vi "Test Reset.vi"(11 "Error in":errorcluster) -> (15 "Error out":errorcluster)   [LabVIEW 2020, in "StopWatchTests.lvlib"]
doc: "This VI is used for validating reset button in stopwatch"
uses:
  StopWatchTests.lvlib
  <vilib>/SLL Drona/APIs/Stimulus/ControlValue/SetValueAuto.vi
  <vilib>/SLL Drona/APIs/Assert/AssertControlValue/Equal.vi
  <vilib>/SLL Drona/APIs/Assert/AssertControlValue/Greater.vi
  <vilib>/SLL Drona/APIs/Stimulus/VI/CloseVI.vi
  <vilib>/addons/_JKI Toolkits/Caraya/classes/Test/Test.lvclass
  <vilib>/SLL Drona/Drona.lvlib
  <vilib>/SLL Drona/APIs/Stimulus/ControlValue/ControlValue.lvlib
  <vilib>/SLL Drona/APIs/Assert/AssertControlValue/AssertControlValue.lvlib
  <vilib>/SLL Drona/APIs/Stimulus/VI/VI.lvlib
panel:
  # "RESET TEST"
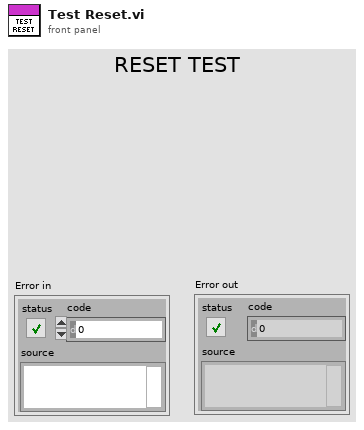
[diagram p1: front panel]
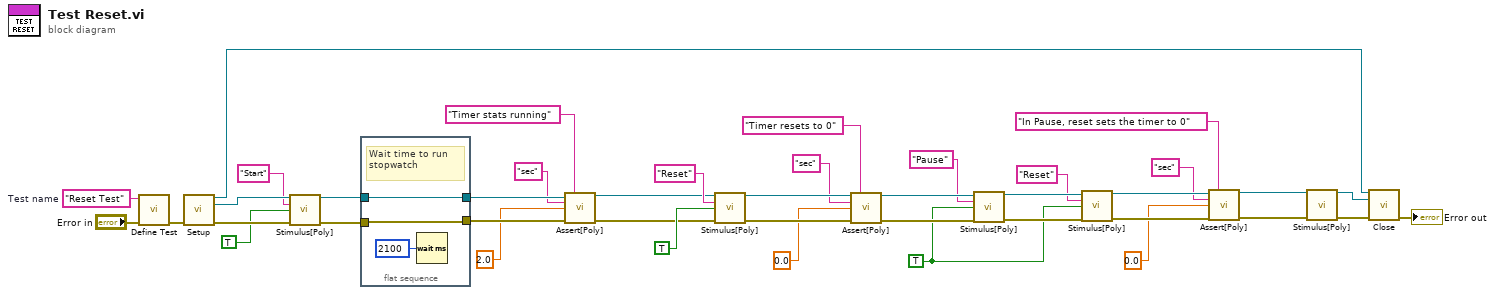
[diagram p0: block diagram]
diagram:
  w8 = TRUE
  w40 = "Reset Test"  # Test name
  n1 = call <vilib>:"Define Test.vi"("error in (no error)"="Error in", "Label (VI Title)"=w40) -> ("error out"=w39:errorcluster)  [unwired: 9 in]
  n2 = call <vilib>:"Setup.vi"("error in"=w39) -> ("Application Ref"=w37:refnum<vi>, "VI Reference Out"=w33:refnum<vi>, "error out"=w34:errorcluster)  [unwired: 12 in]
  n3 = call-poly <vilib>:"Stimulus[Poly].vi"("VI Reference In"=w33, "Control Path"="Start", "Value (Signaling)"=TRUE, "error in"=w34) -> ("VI Reference Out"=w29:refnum<vi>, "error out"=w30:errorcluster)  [unwired: 10 in]
  n4 = flat-sequence {
    tunnel: w30 -> [w43]
    tunnel: [w43] -> w21
    tunnel: w29 -> [w42]
    tunnel: [w42] -> w20
    frame #0 {
      # "Wait time to run  stopwatch"
      n5 = Wait (ms)(milliseconds to wait=u32 2100) -> ()  [unwired: 1 out]
    }
  }
  n6 = call-poly <vilib>:"Assert[Poly].vi"("VI Reference In"=w20, "Test Label"="Timer stats running", "Control Path"="sec", "Control Value"=2.0, "Error In"=w21) -> ("VI Reference Out"=w15:refnum<vi>, "Error Out"=w16:errorcluster)  [unwired: 9 in]
  n7 = call-poly <vilib>:"Stimulus[Poly].vi"("VI Reference In"=w15, "Control Path"="Reset", "Value (Signaling)"=TRUE, "error in"=w16) -> ("VI Reference Out"=w25:refnum<vi>, "error out"=w26:errorcluster)  [unwired: 10 in]
  n8 = call-poly <vilib>:"Assert[Poly].vi"("VI Reference In"=w25, "Test Label"="Timer resets to 0", "Control Path"="sec", "Control Value"=0.0, "Error In"=w26) -> ("VI Reference Out"=w13:refnum<vi>, "Error Out"=w14:errorcluster)  [unwired: 9 in]
  n9 = call-poly <vilib>:"Stimulus[Poly].vi"("VI Reference In"=w13, "Control Path"="Pause", "Value (Signaling)"=w8, "error in"=w14) -> ("VI Reference Out"=w10:refnum<vi>, "error out"=w11:errorcluster)  [unwired: 10 in]
  n10 = call-poly <vilib>:"Stimulus[Poly].vi"("VI Reference In"=w10, "Control Path"="Reset", "Value (Signaling)"=w8, "error in"=w11) -> ("VI Reference Out"=w6:refnum<vi>, "error out"=w7:errorcluster)  [unwired: 10 in]
  n11 = call-poly <vilib>:"Assert[Poly].vi"("VI Reference In"=w6, "Test Label"="In Pause, reset sets the timer to 0", "Control Path"="sec", "Control Value"=0.0, "Error In"=w7) -> ("VI Reference Out"=w1:refnum<vi>, "Error Out"=w2:errorcluster)  [unwired: 9 in]
  n12 = call-poly <vilib>:"Stimulus[Poly].vi"("VI Reference In"=w1, "error in"=w2) -> ("VI Reference Out"=w36:refnum<vi>, "error out"=w35:errorcluster)  [unwired: 12 in]
  n13 = call <vilib>:"Close.vi"("Application Ref"=w37, "VI Reference"=w36, "error in"=w35) -> ("error out"=→"Error out":errorcluster)  [unwired: 12 in]
